vi "Delete Empty Folders Recursively.vi"(4 "Folders to Exclude":string[](array[string]), 8 "error in (no error)":errorcluster, 11 "Folder Path":path=path "C:/temp/TDMS rename") -> (0 "error out":errorcluster)   [LabVIEW 2020]
doc: "This VI will delete all empty folders, under a given folder path.\n\n-------------\nPackage Information\n\nProduct Name: Hooovahh File IO\nPackage File Name: Hooovahh_File_IO\nPackage Version: 1.0.2.4\nMinimum LabVIEW Version: 20.0"
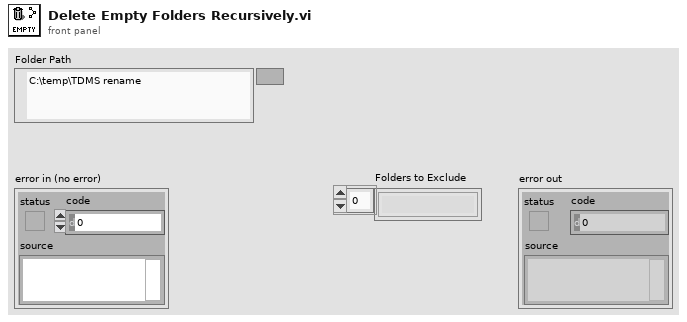
[diagram p1: front panel]
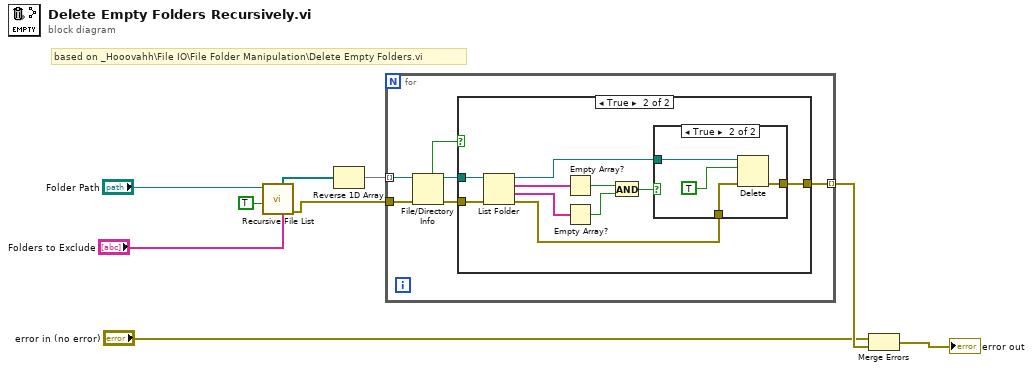
[diagram p0: block diagram]
diagram:
  # "based on _Hooovahh\\File IO\\File Folder Manipulation\\Delete Empty Folders.vi"
  n1 = call <vilib>:"Recursive File List.vi"("Folders to Exclude"="Folders to Exclude", "Continue Recursing on Error? (F)"=TRUE, "Folder Path"="Folder Path") -> ("error out"=w1:errorcluster, "All Folders"=w5:path[])  [unwired: 4 in, 3 out]
  n2 = Reverse 1D Array(array=w5) -> (reversed array=w8:path[])
  n3 = for {
    tunnel: w8 -> [w15] mode=indexing
    tunnel: w1 -> [w12]
    tunnel: [w10] -> w7 mode=indexing
    n4 = File/Directory Info(path=w15, error in=w12) -> (path out=w14:path, directory=w13:bool, error out=w11:errorcluster)  [unwired: 4 out]
    n5 = case shown="True" w13 {
      tunnel: w14 -> [_ w26]
      tunnel: w11 -> [w16 w19]
      tunnel: [w16 w17] -> w10
      frame False {
      }
      frame True {
        n6 = List Folder(path=w26, error in=w19) -> (path out=w23:path, filenames=w25:string[], folder names=w22:string[], error out=w18:errorcluster)  [unwired: 2 in]
        n7 = Empty Array?(array=w25) -> (empty?=w24:bool)
        n8 = Empty Array?(array=w22) -> (empty?=w20:bool)
        n9 = And(x=w24, y=w20) -> (x .and. y?=w21:bool)
        n10 = case shown="True" w21 {
          tunnel: w23 -> [_ w31]
          tunnel: w18 -> [w27 w29]
          tunnel: [w27 w28] -> w17
          frame False {
          }
          frame True {
            n11 = Delete(path (use dialog)=w31, entire hierarchy (F)=TRUE, error in=w29) -> (error out=w28:errorcluster)  [unwired: 2 in, 2 out]
          }
        }
      }
    }
  }
  n12 = Merge Errors("error in (no error)", w7) -> (→"error out":errorcluster)
